vi "Find destination from source.vi"(7 "Connections":T1[](array[typedef]), 11 "Source":i64) -> (3 "Destination":i64, 5 "Offset":i64)   [LabVIEW 2023]
uses:
  Cluster_Sorce Destination Connection.ctl
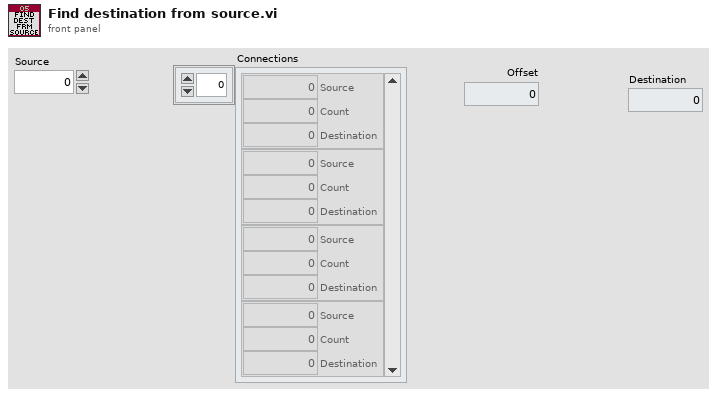
[diagram p1: front panel]
types:
  T1 = typedef "Cluster_Sorce Destination Connection.ctl" = cluster{"Source":i64, "Count":i64, "Destination":i64}
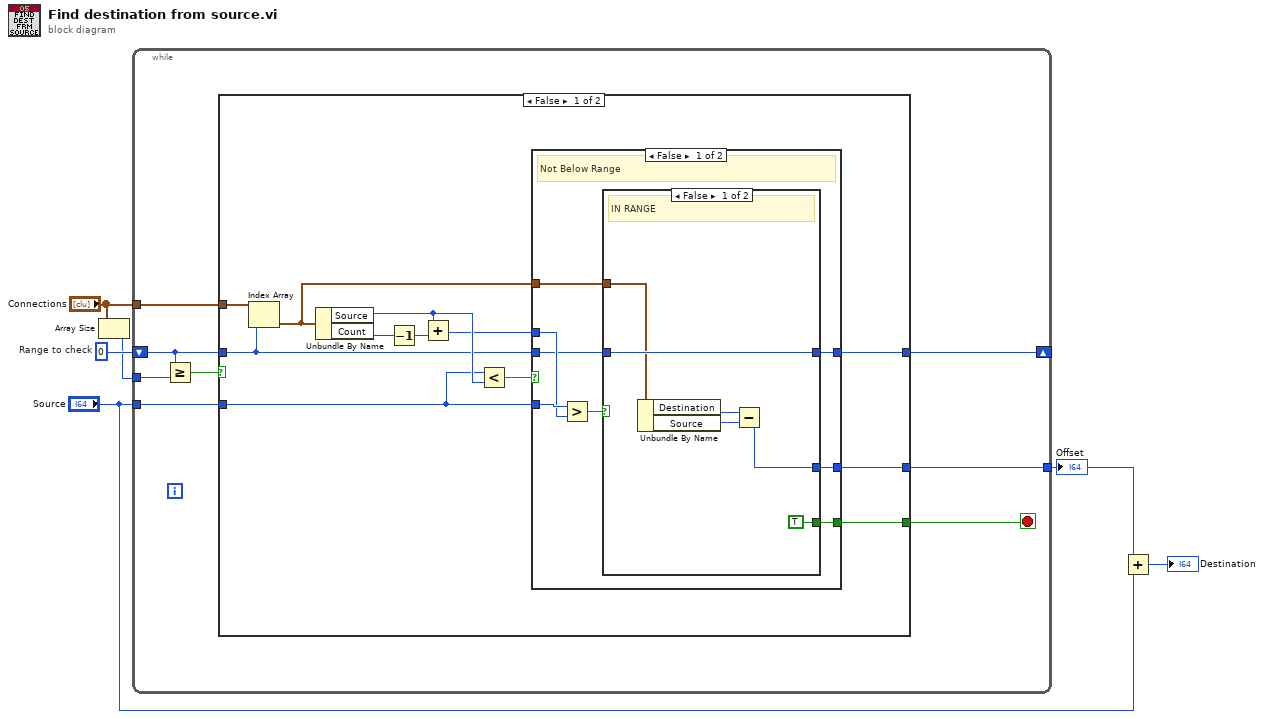
[diagram p0: block diagram]
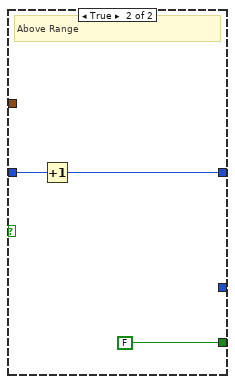
[diagram p2: hidden frame]
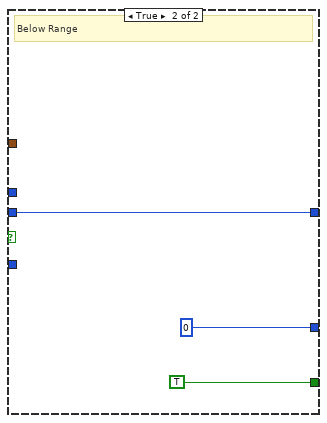
[diagram p3: hidden frame]
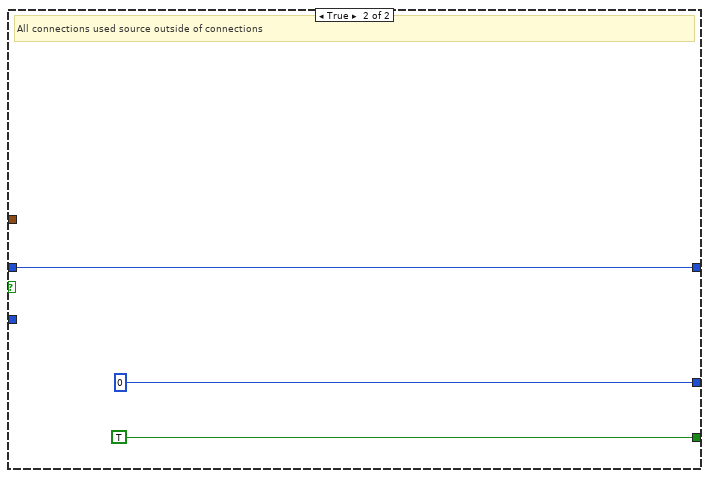
[diagram p4: hidden frame]
diagram:
  w6 = 0  # Range to check
  n1 = Array Size(array="Connections") -> (size(s)=w1:i32)
  n2 = while {
    tunnel: "Source" -> [w11]
    tunnel: "Connections" -> [w14]
    shift-right: [w10] -> _
    shift-left: w6 -> [w9]
    tunnel: [w12] -> w5
    tunnel: w1 -> [w8]
    stop <- w13 stop-if-true
    n3 = Greater Or Equal?(x=w9, y=w8) -> (x >= y?=w7:bool)
    n4 = case shown="False" w7 {
      tunnel: w14 -> [w26 _]
      tunnel: [w21 TRUE] -> w13
      tunnel: [w20 i64 0] -> w12
      tunnel: w11 -> [w18 _]
      tunnel: [w16 w49] -> w10
      tunnel: w9 -> [w15 w49]
      frame False {
        n5 = Index Array(array=w26, index=w15) -> (element=w19:T1)
        n6 = Unbundle By Name(w19) -> ("Source"=w23:i64, "Count"=w25:i64)
        n7 = Decrement(x=w25) -> (x-1=w24:i64)
        n8 = Add(x=w23, y=w24) -> (x+y=w17:i64)
        n9 = Less?(x=w18, y=w23) -> (x < y?=w22:bool)
        n10 = case shown="False" w22 {
          tunnel: w15 -> [w30 w44]
          tunnel: [w31 TRUE] -> w21
          tunnel: [w27 i64 0] -> w20
          tunnel: w19 -> [w28 _]
          tunnel: w18 -> [w34 _]
          tunnel: w17 -> [w33 _]
          tunnel: [w29 w44] -> w16
          frame False {
            # "Not Below Range"
            n11 = Greater?(x=w34, y=w33) -> (0:w32:bool)
            n12 = case shown="False" w32 {
              tunnel: [TRUE FALSE] -> w31
              tunnel: w30 -> [w40 w42]
              tunnel: [w40 w41] -> w29
              tunnel: w28 -> [w39 _]
              tunnel: [w36 _] -> w27
              frame False {
                # "IN RANGE"
                n13 = Unbundle By Name(w39) -> ("Destination"=w38:i64, "Source"=w37:i64)
                n14 = Subtract(x=w38, y=w37) -> (x-y=w36:i64)
              }
              frame True {
                # "Above Range"
                n15 = Increment(x=w42) -> (x+1=w41:i32)
              }
            }
          }
          frame True {
            # "Below Range"
          }
        }
      }
      frame True {
        # "All connections used source outside of connections"
      }
    }
  }
  "Offset" <- w5
  n16 = Add(x=w5, y="Source") -> (x+y=→"Destination":i64)
